vi "GetWaveformGraphReference.vi"(8 "error in":errorcluster, 11 "WFGraph in":refnum<class "WaveformGraph.lvclass">) -> (0 "error out":errorcluster, 1 "WFGraph reference":refnum<vi>, 3 "WFGraph out":refnum<class "WaveformGraph.lvclass">)   [LabVIEW 2014, in "WaveformGraph.lvclass"]
uses:
  WaveformGraph.lvclass
  Generic/Generic.lvclass
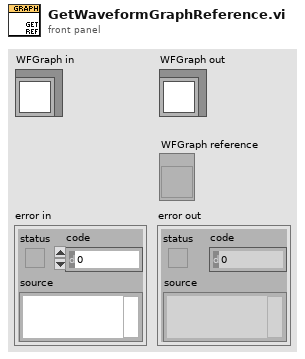
[diagram p1: front panel]
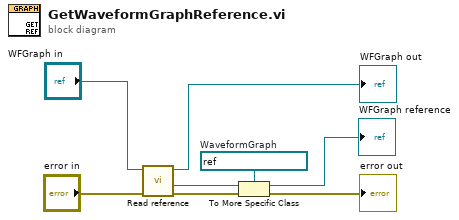
[diagram p0: block diagram]
diagram:
  w5 = refnum<vi> refnum  # WaveformGraph
  n1 = call "Read reference.vi"("error in"="error in", "GObject in"="WFGraph in") -> ("error out"=w6:errorcluster, "reference"=w7:refnum<vi>, "GObject out"=→"WFGraph out":refnum<class "WaveformGraph.lvclass">)  [unwired: 5 in]
  n2 = To More Specific Class(target class=w5, reference=w7, error in=w6) -> (specific class reference=→"WFGraph reference":refnum<vi>, error out=→"error out":errorcluster)
